vi "kanaly to array.vi"(10 "Kanaly":T1) -> (0 "Rozmiar":u32, 2 "Kanaly Array":waveform(dbl)[](array[waveform]))   [LabVIEW 2013]
uses:
  Kontrolki/Przetwarzanie/Kanaly.ctl
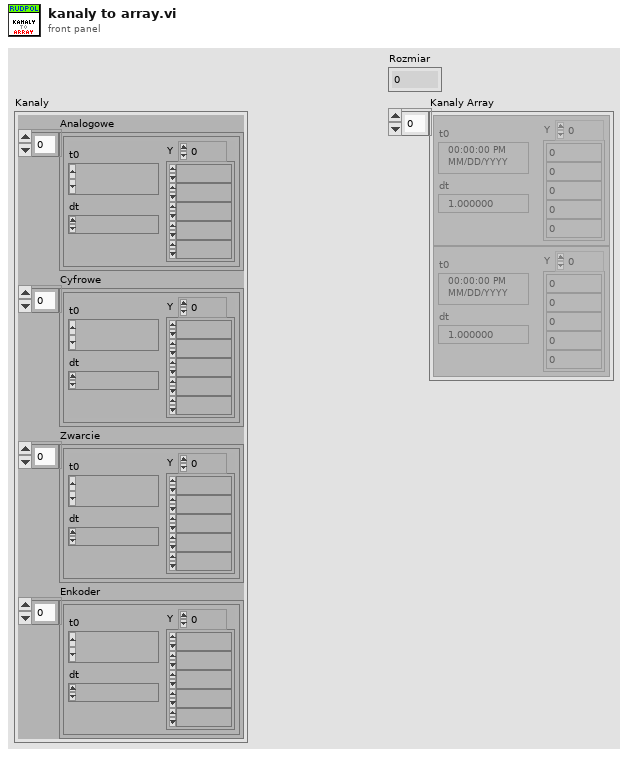
[diagram p1: front panel]
types:
  T1 = typedef "Kanaly.ctl" = cluster{"Analogowe":waveform(dbl)[], "Cyfrowe":waveform(dbl)[], "Zwarcie":waveform(dbl)[], "Enkoder":waveform(dbl)[]}
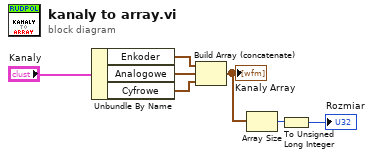
[diagram p0: block diagram]
diagram:
  n1 = Unbundle By Name("Kanaly") -> ("Enkoder"=w5:waveform(dbl)[], "Analogowe"=w6:waveform(dbl)[], "Cyfrowe"=w7:waveform(dbl)[])
  n2 = Build Array (concatenate)(w5, w6, w7) -> (w2:waveform(dbl)[])
  "Kanaly Array" <- w2
  n3 = Array Size(array=w2) -> (size(s)=w3:i32)
  n4 = To Unsigned Long Integer(number=w3) -> (unsigned 32bit integer=→"Rozmiar":u32)
